vi "DAQmx Create Channel (CI-Pulse Freq).vi"(0 "task in":refnum<k21>, 1 "maximum value":dbl=1000000.0 format="%.6f", 2 "minimum value":dbl=1000.0 format="%.6f", 5 "counter":tag, 7 "name to assign":string, 9 "units":i32(ring)=10373 items=["Hz"=10373], 11 "error in":errorcluster) -> (4 "task out":refnum<k21>, 15 "error out":errorcluster)   [LabVIEW 2011]
doc: "Creates a channel to measure pulse specifications, returning the measurements as pairs of frequency and duty cycle. You can create only one counter input channel at a time with this VI because a task can contain only one counter input channel. To read from multiple counters simultaneously, use a separate task for each counter. Connect the input signal to the default input terminal of the counter unless you select a different input terminal."
uses:
  C:/Program Files/National Instruments/LabVIEW 2011/resource/objmgr/daqmx.rc
panel:
  # "input limits"
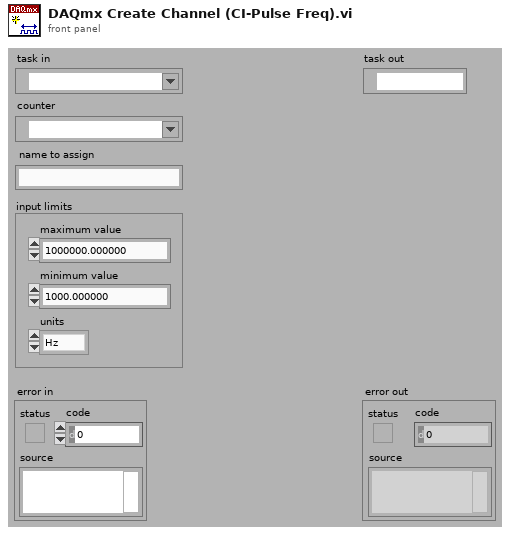
[diagram p1: front panel]
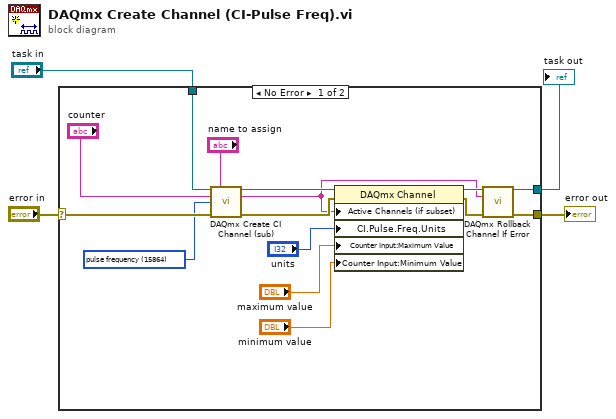
[diagram p0: block diagram]
diagram:
  n1 = case shown="No Error" "error in" {
    selector: "error in" -> [w18 w20]
    tunnel: "task in" -> [w19 w21]
    tunnel: [w10 w21] -> w2
    tunnel: [w9 w20] -> w1
    frame No Error {
      w6 = 15864 items=["count events"=10125, "frequency"=10179, "period"=10256, "pulse width"=10359, "semi period"=10289, "pulse frequency"=15864, "pulse time"=15865, "pulse ticks"=15866, "two edge separation"=10267, "angular encoder"=10360, "linear encoder"=10361, "gps timestamp"=10362] ("measurement type")
      n2 = call "DAQmx Create CI Channel (sub).vi"("task in"=w19, "virtual channel name"="name to assign", "physical channel name"="counter", "measurement type"=w6, "error in"=w18) -> ("task out"=w14:refnum<k21>, "channel names"=w7:string, "error out"=w16:errorcluster)  [unwired: 1 in, 7 out]
      n3 = property class="DAQmx Channel"(reference=w14, error in=w16, "Active Channels (if subset)"=w7, "CI.Pulse.Freq.Units"="units", "Counter Input:Maximum Value"="maximum value", "Counter Input:Minimum Value"="minimum value") -> (reference out=w11:refnum<k21>, error out=w8:errorcluster)
      n4 = call "DAQmx Rollback Channel If Error.vi"("task in"=w11, "channel names"=w7, "error in"=w8) -> ("task out"=w10:refnum<k21>, "error out"=w9:errorcluster)  [unwired: 11 out]
    }
    frame Error {
    }
  }
  "error out" <- w1
  "task out" <- w2
